vi "MonkeyType.vi"() -> (0 "Random Character":string)   [LabVIEW 2015]
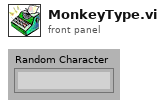
[diagram p1: front panel]
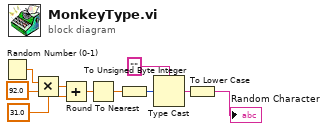
[diagram p0: block diagram]
diagram:
  n1 = Random Number (0-1)() -> (number: 0 to 1=w1:dbl)
  n2 = Multiply(x=w1, y=92.0) -> (x*y=w6:dbl)
  n3 = Add(x=w6, y=31.0) -> (x+y=w8:dbl)
  n4 = Round To Nearest(number=w8) -> (nearest integer value=w3:dbl)
  n5 = To Unsigned Byte Integer(number=w3) -> (unsigned 8bit integer=w4:u8)
  n6 = Type Cast(type="", x=w4) -> (*(type *) &x=w9:string)
  n7 = To Lower Case(string=w9) -> (all lower case string=→"Random Character":string)
